vi "PWM.vi"(10 "Duty Cycle":fxp<+,32,0>, 11 "Period (Ticks)":u32) -> (0 "Count":u32, 3 "PWM Out":bool)   [LabVIEW 2016, in "jmslib.lvlib"]
uses:
  jmslib.lvlib
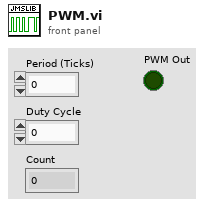
[diagram p1: front panel]
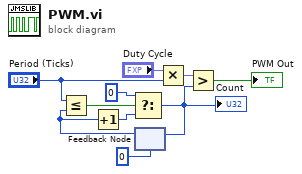
[diagram p0: block diagram]
diagram:
  n1 = feedback #1(u32 0) -> (w9:u32)
  n2 = Less Or Equal?(x="Period (Ticks)", y=w9) -> (x <= y?=w3:bool)
  n3 = Increment(x=w9) -> (x+1=w6:u32)
  n4 = Select(t=u32 0, s=w3, f=w6) -> (s? t:f=w4:u32)
  "Count" <- w4
  n5 = feedback-in #1(w4) -> ()
  n6 = Multiply(x="Duty Cycle", y="Period (Ticks)") -> (x*y=w7:fxp<+,64,32>)
  n7 = Greater?(x=w7, y=w4) -> (0:→"PWM Out":bool)
